vi "Process harness.vi"() -> ()   [LabVIEW 2013, in "LED tests.lvlib"]
uses:
  LED tests.lvlib
  module/execution/parameter user data.ctl
  module/execution/LED runtime.lvclass
panel:
  in  "Parameters to process":T1={"Enable"=FALSE, "Blinks per cycle"=0, "Green (T) Yellow (F)"=FALSE, "Blink period (s)"=1.0}
  in  "stop":bool
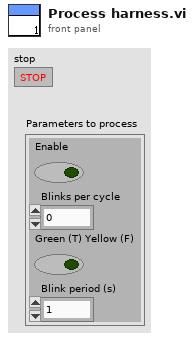
[diagram p1: front panel]
types:
  T1 = typedef "LED runtime.lvclass/parameter user data.ctl" = cluster{"Enable":bool, "Blinks per cycle":i32, "Green (T) Yellow (F)":bool, "Blink period (s)":dbl}
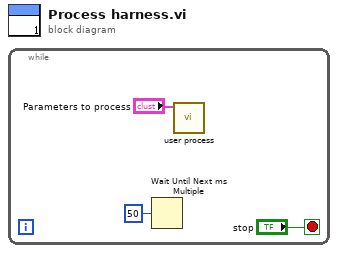
[diagram p0: block diagram]
diagram:
  n1 = while {
    stop <- "stop" stop-if-true
    n2 = Wait Until Next ms Multiple(millisecond multiple=u32 50) -> ()  [unwired: 1 out]
    n3 = call "user process.vi"("Parameters to process"="Parameters to process") -> ()  [unwired: 9 in, 2 out]
  }
